vi "StateSpace_WalkThrough_Example.vi"() -> ()   [LabVIEW 2019]
uses:
  <vilib>/Rock Robotics/WPI/ThirdParty/JAS_Junk/TrajLib/TypeDef/LINEAR_SYSTEM.ctl
  <vilib>/Analysis/Matrix/Datatypes/RealMatrix.ctl
  <vilib>/Rock Robotics/WPI/ThirdParty/JAS_Junk/TrajLib/TypeDef/DCMOTOR.CTL
  <vilib>/Rock Robotics/WPI/ThirdParty/JAS_Junk/TrajLib/TypeDef/LINEAR_QUADRATIC_REGULATOR.ctl
  <vilib>/Rock Robotics/WPI/ThirdParty/JAS_Junk/TrajLib/TypeDef/KALMAN_FILTER.ctl
  <vilib>/Rock Robotics/WPI/ThirdParty/JAS_Junk/TrajLib/TypeDef/LINEAR_SYSTEM_LOOP.ctl
  <vilib>/Rock Robotics/WPI/ThirdParty/JAS_Junk/TrajLib/TypeDef/LINEAR_PLANT_INV_FF.ctl
  <vilib>/Rock Robotics/WPI/ThirdParty/JAS_Junk/TrajLib/TypeDef/FLYWHEEL_SIM.ctl
  <vilib>/Rock Robotics/WPI/ThirdParty/JAS_Junk/TrajLib/TypeDef/LINEAR_SYSTEM_SIM.ctl
  <vilib>/Rock Robotics/WPI/ThirdParty/JAS_Junk/TrajLib/Enum/DCMOTOR_TYPES_ENUM.ctl
  <vilib>/Rock Robotics/WPI/ThirdParty/JAS_Junk/TrajLib/DCMotor_GetCIM.vi
  <vilib>/Rock Robotics/WPI/ThirdParty/JAS_Junk/TrajLib/DCMotor_GetAndymark9015.vi
  <vilib>/Rock Robotics/WPI/ThirdParty/JAS_Junk/TrajLib/DCMotor_GetAndymarkRs775_125.vi
  <vilib>/Rock Robotics/WPI/ThirdParty/JAS_Junk/TrajLib/DCMotor_GetBag.vi
  <vilib>/Rock Robotics/WPI/ThirdParty/JAS_Junk/TrajLib/DCMotor_GetBanebotsRs550.vi
  <vilib>/Rock Robotics/WPI/ThirdParty/JAS_Junk/TrajLib/DCMotor_GetBanebotsRs775.vi
  <vilib>/Rock Robotics/WPI/ThirdParty/JAS_Junk/TrajLib/DCMotor_GetFalcon500.vi
  <vilib>/Rock Robotics/WPI/ThirdParty/JAS_Junk/TrajLib/DCMotor_GetMiniCIM.vi
  <vilib>/Rock Robotics/WPI/ThirdParty/JAS_Junk/TrajLib/DCMotor_GetNEO.vi
  <vilib>/Rock Robotics/WPI/ThirdParty/JAS_Junk/TrajLib/DCMotor_GetNEO550.vi
  <vilib>/Rock Robotics/WPI/ThirdParty/JAS_Junk/TrajLib/DCMotor_GetRomiBuiltIn.vi
  <vilib>/Rock Robotics/WPI/ThirdParty/JAS_Junk/TrajLib/DCMotor_GetVex775Pro.vi
  <vilib>/Rock Robotics/WPI/ThirdParty/JAS_Junk/TrajLib/MatBuilder_Create.vi
  <vilib>/Rock Robotics/WPI/ThirdParty/JAS_Junk/TrajLib/LinearSystem_New.vi
  <vilib>/Rock Robotics/WPI/ThirdParty/JAS_Junk/TrajLib/MatrixHelper_Zero.vi
  <vilib>/Rock Robotics/WPI/ThirdParty/JAS_Junk/TrajLib/MatBuilder_Fill.vi
  <vilib>/Rock Robotics/WPI/ThirdParty/JAS_Junk/TrajLib/Matrix_Ident.vi
  <vilib>/Rock Robotics/WPI/ThirdParty/JAS_Junk/TrajLib/LinearFilter_ResetToValue.vi
  <vilib>/Rock Robotics/WPI/ThirdParty/JAS_Junk/TrajLib/LinearFilter_Calculate.vi
  <vilib>/Rock Robotics/WPI/ThirdParty/JAS_Junk/TrajLib/DCMotor_New.vi
  <vilib>/Rock Robotics/WPI/ThirdParty/JAS_Junk/TrajLib/VI/Units_RotationsPerMinuteToRadiansPerSecond.vi
  <vilib>/Rock Robotics/WPI/ThirdParty/JAS_Junk/TrajLib/MatrixHelper_CoerceSize.vi
  <vilib>/Analysis/7linalg.llb/Create Special Matrix.vi
  <vilib>/Analysis/7linalg.llb/Create Special Real Matrix.vi
  <vilib>/Rock Robotics/WPI/ThirdParty/JAS_Junk/TrajLib/LinearFilter_MovingAverage.vi
  <vilib>/Rock Robotics/WPI/ThirdParty/JAS_Junk/TrajLib/LinearFilter_LowPassBW1.vi
  <vilib>/Rock Robotics/WPI/ThirdParty/JAS_Junk/TrajLib/LinearFilter_LowPassBW2.vi
  <vilib>/Rock Robotics/WPI/ThirdParty/JAS_Junk/TrajLib/LinearFilter_HighPassBW1.vi
  <vilib>/Rock Robotics/WPI/ThirdParty/JAS_Junk/TrajLib/LinearFilter_HighPassBW2.vi
  <vilib>/Rock Robotics/WPI/ThirdParty/JAS_Junk/TrajLib/Trajectory_Library.lvlib
  <vilib>/Analysis/Matrix/NI_Matrix.lvlib
panel:
  out "Linear System Loop":T1
  in  "Tab Control":T7(tab)
  out "m_flywheelPlant":T6
  out "Error\nSize Coerced":bool
  out "Shooter Motor":T8 {"Jr_KgM2" format="%13.5p"; "L_H" format="%13.5p"; "Kt_NMPerAmp" format="%13.5p"; "KvINV_RadPerSecPerVolt" format="%13.5p"; "R_Ohms" format="%13.5p"; "FreeSpeed_RadPerSec" format="%13.5p"; "FreeCurrent_Amps" format="%13.5p"; "StallCurrent_Amps" format="%13.5p"; "StallTorque_NM" format="%13.5p"; "nominalVoltage_Volts" format="%13.5p"}
  out "m_flywheelPlant_ALT":T6
  out "KalmanFilter":T5
  out "Kalman Creation Error":errorcluster
  out "LinearQuadraticRegulator":T2
  out "LQR Creation Error":bool
  out "Linear System Loop":T1
  out "LinSysLoop_Error":bool
  out "CO, Filtered Voltage, Filtered Current Chart":T9(graph)
  out "Filtereed Battery Voltage":dbl format="%20.3f"
  out "Filtereed Current (Amps)":dbl format="%20.3f"
  in  "Shooter \nOn/Off":bool
  out "Encoder Speed\nRad/Sec":dbl(slide) scale=0.0..300.0
  out "Speed \nRad/Sec":dbl format="%16.1f"
  out "Execution\nError":bool
  out "Kalman Filtered\nSpeed Rad/Sec":dbl format="%16.1f"
  out "SP, PV Chart":T9(graph)
  out "Motor Dmd CO":dbl format="%20.3f"
  out "Speed Setpoint\nRad/Sec":dbl format="%16.1f"
  in  "Set Point\nRad/Sec 2":dbl(slide) scale=0.0..300.0
  out "m_FlyWheelSim":T10 {"GearBox"."Jr_KgM2" format="%13.5p"; "GearBox"."L_H" format="%13.5p"; "GearBox"."Kt_NMPerAmp" format="%13.5p"; "GearBox"."KvINV_RadPerSecPerVolt" format="%13.5p"; "GearBox"."R_Ohms" format="%13.5p"; "GearBox"."FreeSpeed_RadPerSec" format="%13.5p"; "GearBox"."FreeCurrent_Amps" format="%13.5p"; "GearBox"."StallCurrent_Amps" format="%13.5p"; "GearBox"."StallTorque_NM" format="%13.5p"; "GearBox"."nominalVoltage_Volts" format="%13.5p"}
  # "<States,1>"
  # "<FUTURE --- CLAMP TYPE -- For now\nuse Normalize>"
  # "Steady State Gain  \n<States,Outputs>"
  # "State Estimate <Statess,1>"
  # "<States,States>"
  # "<States,Inputs>"
  # "<Outputs,States>"
  # "<Outputs,Inputs>"
  # "<States,1>"
  # "<Inputs,1>"
  # "<States,Inputs>"
  # "<States,States>"
  # "Ref State <States,1>"
  # "Comp and capped \noutput <Inputs,1>"
  # "Controller gain\n<Inputs,States>"
  # "The \"plant\" holds a state-space model of our flywheel. This system has the following properties:\n\n   -  States: [velocity], in radians per second.\n   -  Inputs (what we can \"put in\"): [voltage], in volts.\n   -  Outputs (what we can measure): [velocity], in radians per second.\n\nThere are also constants describing how the system behaves.  For our system these are:\n    Kv ---  Volts per (radian per second)\n    Ka --- Volts per (radian per second squared)\n\n One way the Kv and Ka constants can be found by using the FRC Characterization toolsuite.  \n\nNOTE:\n    Constants were changed to create a more realistic simulation."
  # "<States,States>"
  # "<States,Inputs>"
  # "<Outputs,States>"
  # "<Outputs,Inputs>"
  # "Another way to create a linear system is to use the \"helpers\" available for certain types of systems.\n\nThis uses the following contants:\n   -  DcMotor   --  model cooeficients for a pariticular number of a particular model of motor.\n   -  kFlywheelMomentOfInertia = 0.00032    --    kg * m^2\n   -  kFlywheelGearing = 1.0    --  Reduction between motors and encoder, \n                                     as output over input. If the flywheel spins slower than\n                                     the motors, this number should be greater than one.\n\nThe plant holds a state-space model of our flywheel. This system has the following properties:\n   -  States: [velocity], in radians per second.\n   -  Inputs (what we can \"put in\"): [voltage], in volts.\n   -  Outputs (what we can measure): [velocity], in radians per second.\n\nNOTE:\n    Constants were changed to create a more realistic simulation."
  # "<States,States>"
  # "<States,Inputs>"
  # "<Outputs,States>"
  # "<Outputs,Inputs>"
  # "Create a Kalman Filter.  This filters the measurment data, by using the \nLinear System model and how accurate we think the model and \nmeasurements are.  \n\nThe parameters are:\n   - States  --  Number of states in the Linear System\n   - Outputs  --  Number of outputs in the Linear System.\n   - State Std Dev  --  How accurate we think our model is\n   - Measurement Std Dev  --  How accurate we think our encoder data is\n   - dtSeconds  --  How often the control loop will be executed.\n\nNOTE:\n    Constants were changed to create a more realistic simulation."
  # "Steady State Gain  \n<States,Outputs>"
  # "State Estimate <Statess,1>"
  # "<States,States>"
  # "<States,Inputs>"
  # "<Outputs,States>"
  # "<Outputs,Inputs>"
  # "Create the Linear Quadratic Controller.   This takes the measurement input (filtered or not), the desired\nsetpoint (Next R) and calculates the desired motor demand output  U. (Linear System Input) .\n\nCreation of the Linear Quadratic Controller (LQR) takes the following inputs:\n\n   - The Linear System model\n   - Qelms  --  Velocity error tolerance, in radians per second. Decrease\n                         this to more heavily penalize state excursion, or make the controller \n                          behave more aggressively.\n   - Relms  --  Control effort (voltage) tolerance. Decrease this to more\n                        heavily penalize control effort, or make the controller less \n                        aggressive. 12 is a good starting point because that is the \n                        (approximate) maximum voltage of a battery.\n   - dtSeconds  --  Nominal time between loops."
  # "Ref State <States,1>"
  # "Comp and capped \noutput <Inputs,1>"
  # "Controller gain\n<Inputs,States>"
  # "Put everything created so far together into\na Linear System Loop.  This is a convience\nfunction used to help simplify run-time\nexecution."
  # "<States,1>"
  # "<FUTURE --- CLAMP TYPE -- For now\nuse Normalize>"
  # "Steady State Gain  \n<States,Outputs>"
  # "State Estimate <Statess,1>"
  # "<States,States>"
  # "<States,Inputs>"
  # "<Outputs,States>"
  # "<Outputs,Inputs>"
  # "<States,1>"
  # "<Inputs,1>"
  # "<States,Inputs>"
  # "<States,States>"
  # "Ref State <States,1>"
  # "Comp and capped \noutput <Inputs,1>"
  # "Controller gain\n<Inputs,States>"
  # "This subVI is called from a loop that runs every\n20 milliseconds.  The single execution loop with\nshift register in the subVI allows the linear system\nloop state to be saved between calls."
  # "The execution steps are:\n\n1) Set the speed setpoint.\n\n2) Feed the current encoder speed measurement to the \n    controller\n\n3) Execute \"Correct\".  In this step the Kalman filter updates \n    the system state vector with the filtered encoder data.\n\n4) Execute \"Predict\".  This updates the LQR controller to \n    generate new voltage commands and use the voltages \n    to predict the next state with out Kalman filter.\n\n5) Get the desirec motor demand.  This is volts.  It needs \n    to be scaled to +/- 1.0 by dividing by 12.0 to send to the \n    motor controller."
  # "This simulates the Flywheel so the encoder speed can\nbe obtained for this example."
  # "<States, 1>"
  # "<Outputs, 1>"
  # "<Inputs, 1>"
  # "<Outputs, 1>"
  # "<States,States>"
  # "<States,Inputs>"
  # "<Outputs,States>"
  # "<Outputs,Inputs>"
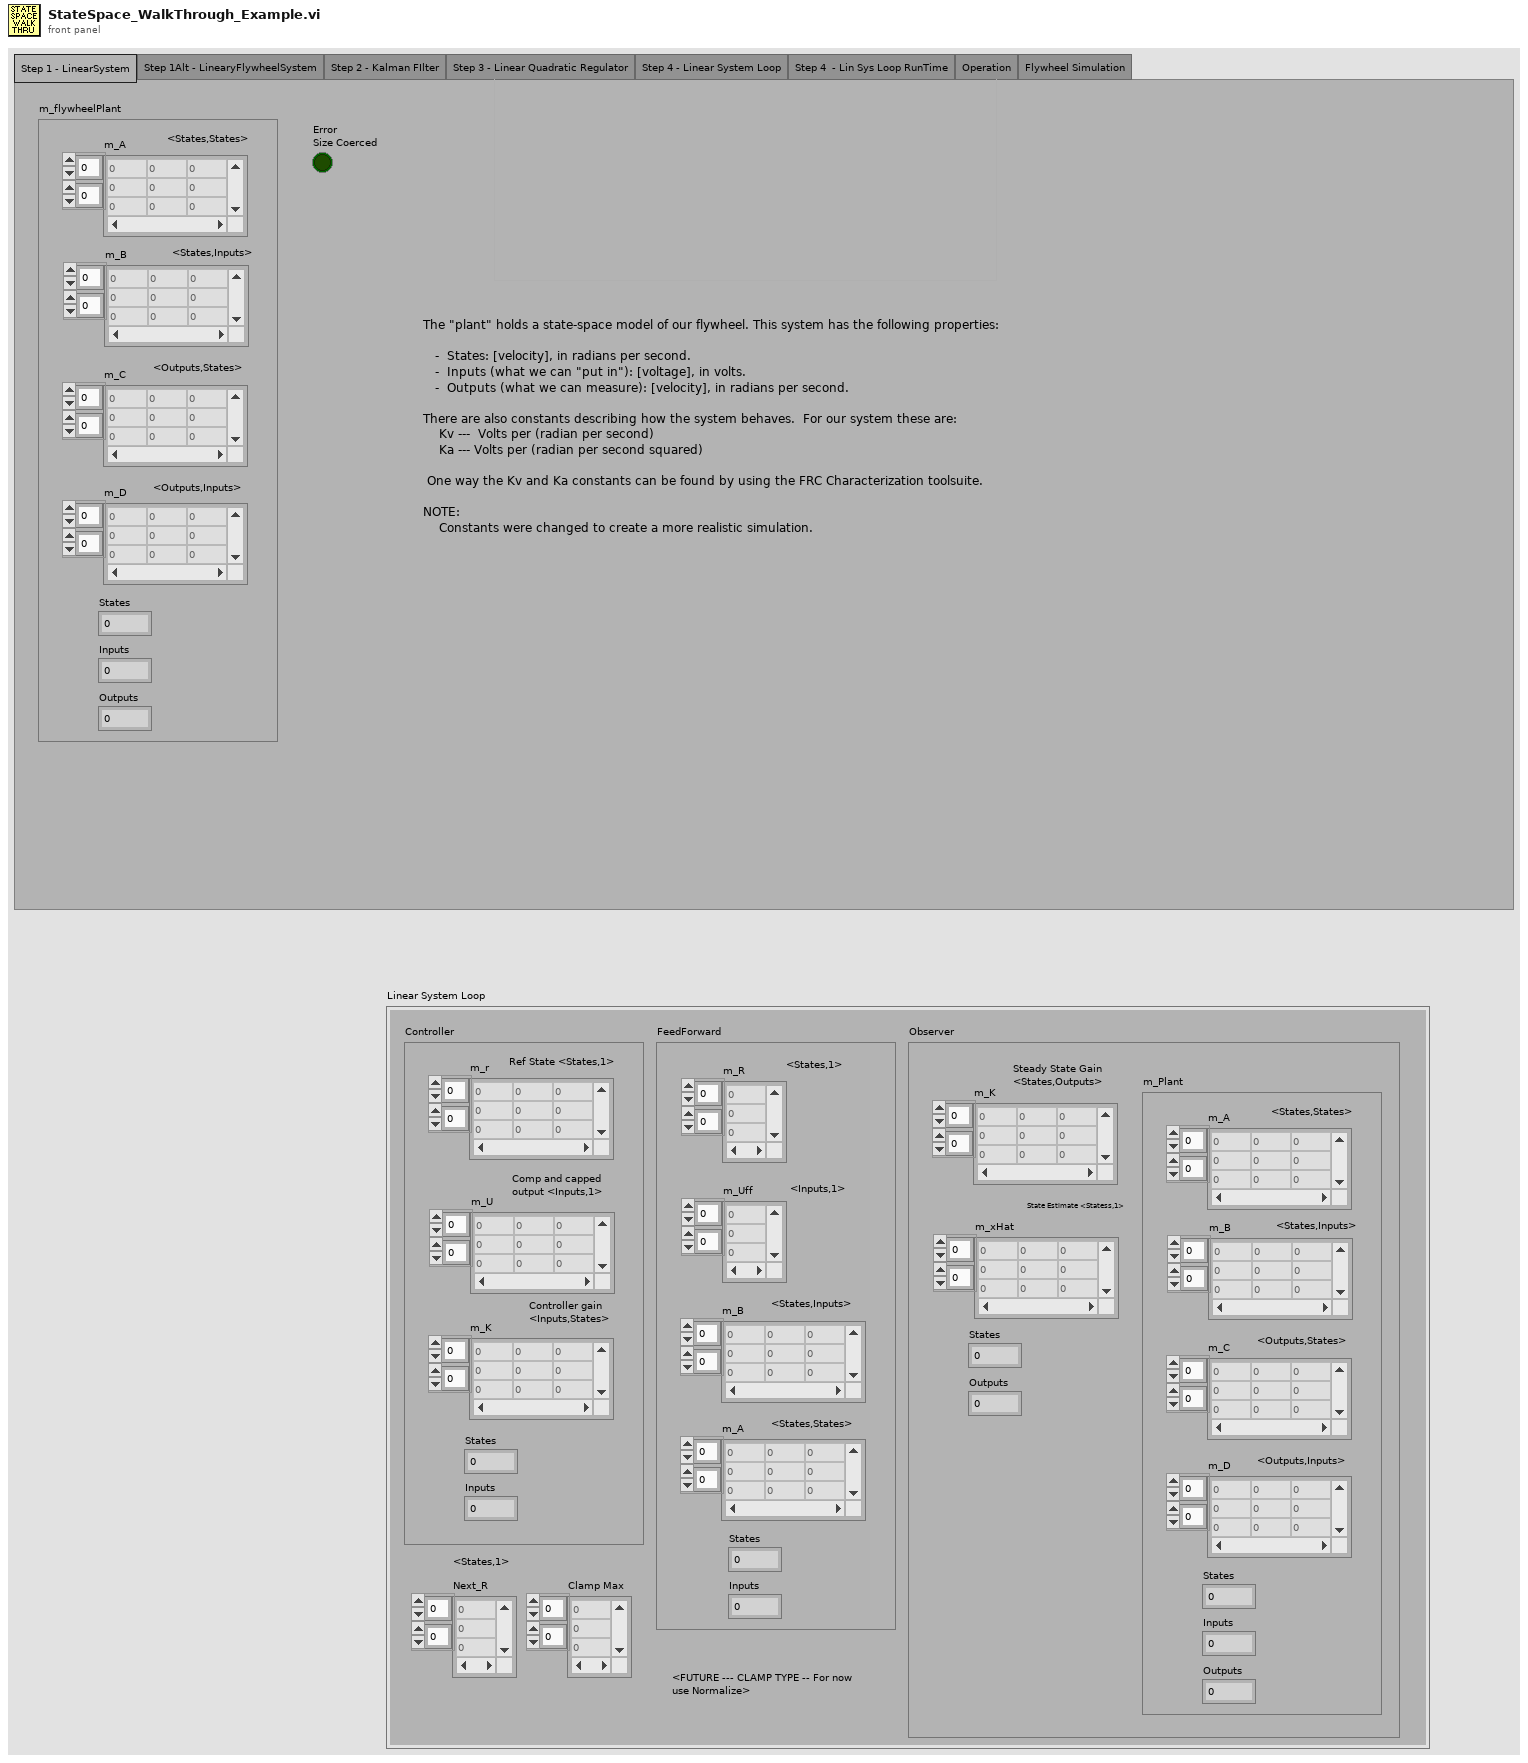
[diagram p1: front panel]
types:
  T1 = typedef "Trajectory_Library.lvlib/LINEAR_SYSTEM_LOOP.ctl" = cluster{"Controller":T2, "FeedForward":T4, "Observer":T5, "Next_R":T3, "Clamp Max":T3}
  T2 = typedef "Trajectory_Library.lvlib/LINEAR_QUADRATIC_REGULATOR.ctl" = cluster{"m_r":T3, "m_U":T3, "m_K":T3, "States":i32, "Inputs":i32}
  T3 = typedef "NI_Matrix.lvlib/RealMatrix.ctl" = dbl[][]
  T4 = typedef "Trajectory_Library.lvlib/LINEAR_PLANT_INV_FF.ctl" = cluster{"m_R":T3, "m_Uff":T3, "m_B":T3, "m_A":T3, "States":i32, "Inputs":i32}
  T5 = typedef "Trajectory_Library.lvlib/KALMAN_FILTER.ctl" = cluster{"m_K":T3, "m_xHat":T3, "States":i32, "Outputs":i32, "m_Plant":T6}
  T6 = typedef "Trajectory_Library.lvlib/LINEAR_SYSTEM.ctl" = cluster{"m_A":T3, "m_B":T3, "m_C":T3, "m_D":T3, "States":i32, "Inputs":i32, "Outputs":i32}
  T7 = enum32{"Step 1 - LinearSystem", "Step 1Alt - LinearyFlywheelSystem", "Step 2 - Kalman FIlter", "Step 3 - Linear Quadratic Regulator", "Step 4 - Linear System Loop", "Step 4  - Lin Sys Loop RunTime", "Operation", "Flywheel Simulation"}
  T8 = typedef "Trajectory_Library.lvlib/DCMOTOR.CTL" = cluster{"nominalVoltage_Volts":dbl, "StallTorque_NM":dbl, "StallCurrent_Amps":dbl, "FreeCurrent_Amps":dbl, "FreeSpeed_RadPerSec":dbl, "R_Ohms":dbl, "KvINV_RadPerSecPerVolt":dbl, "Kt_NMPerAmp":dbl, "L_H":dbl, "Jr_KgM2":dbl}
  T9 = cluster{"upper limit":dbl, "Real Matrix Element":dbl, "Real Matrix Element":dbl}
  T10 = typedef "Trajectory_Library.lvlib/FLYWHEEL_SIM.ctl" = cluster{"LinearSystemSim":T11, "GearBox":T8, "Gearing":dbl}
  T11 = typedef "Trajectory_Library.lvlib/LINEAR_SYSTEM_SIM.ctl" = cluster{"m_Plant":T6, "m_X":T3, "m_Y":T3, "m_U":T3, "MeasureStdDev":T3}
  T12 = typedef "Trajectory_Library.lvlib/DCMOTOR_TYPES_ENUM.ctl" = enum16{"CIM", "AndyMark 9015", "Andy Mark RS 775 125", "Bag", "BaneBots RS 550", "BaneBots RS 775", "Falcon 500", "Mini CIM", "NEO", "NEO 550", "Romi BuiltIn", "Vex 775 Pro"}
  T13 = enum16{"Moving Average", "Low Pass 1st Order Butterworth", "Low Pass 2nd Order Butterworth", "High Pass 1st Order Butterworth", "High Pass 2nd Order Butterworth"}
  T14 = cluster{"Speed Rad/Sec\nPV":dbl, "Filtered PV":dbl, "R0_C0":dbl}
  T15 = cluster{"Motor Dmd CO":dbl, "Output":dbl, "Output":dbl}
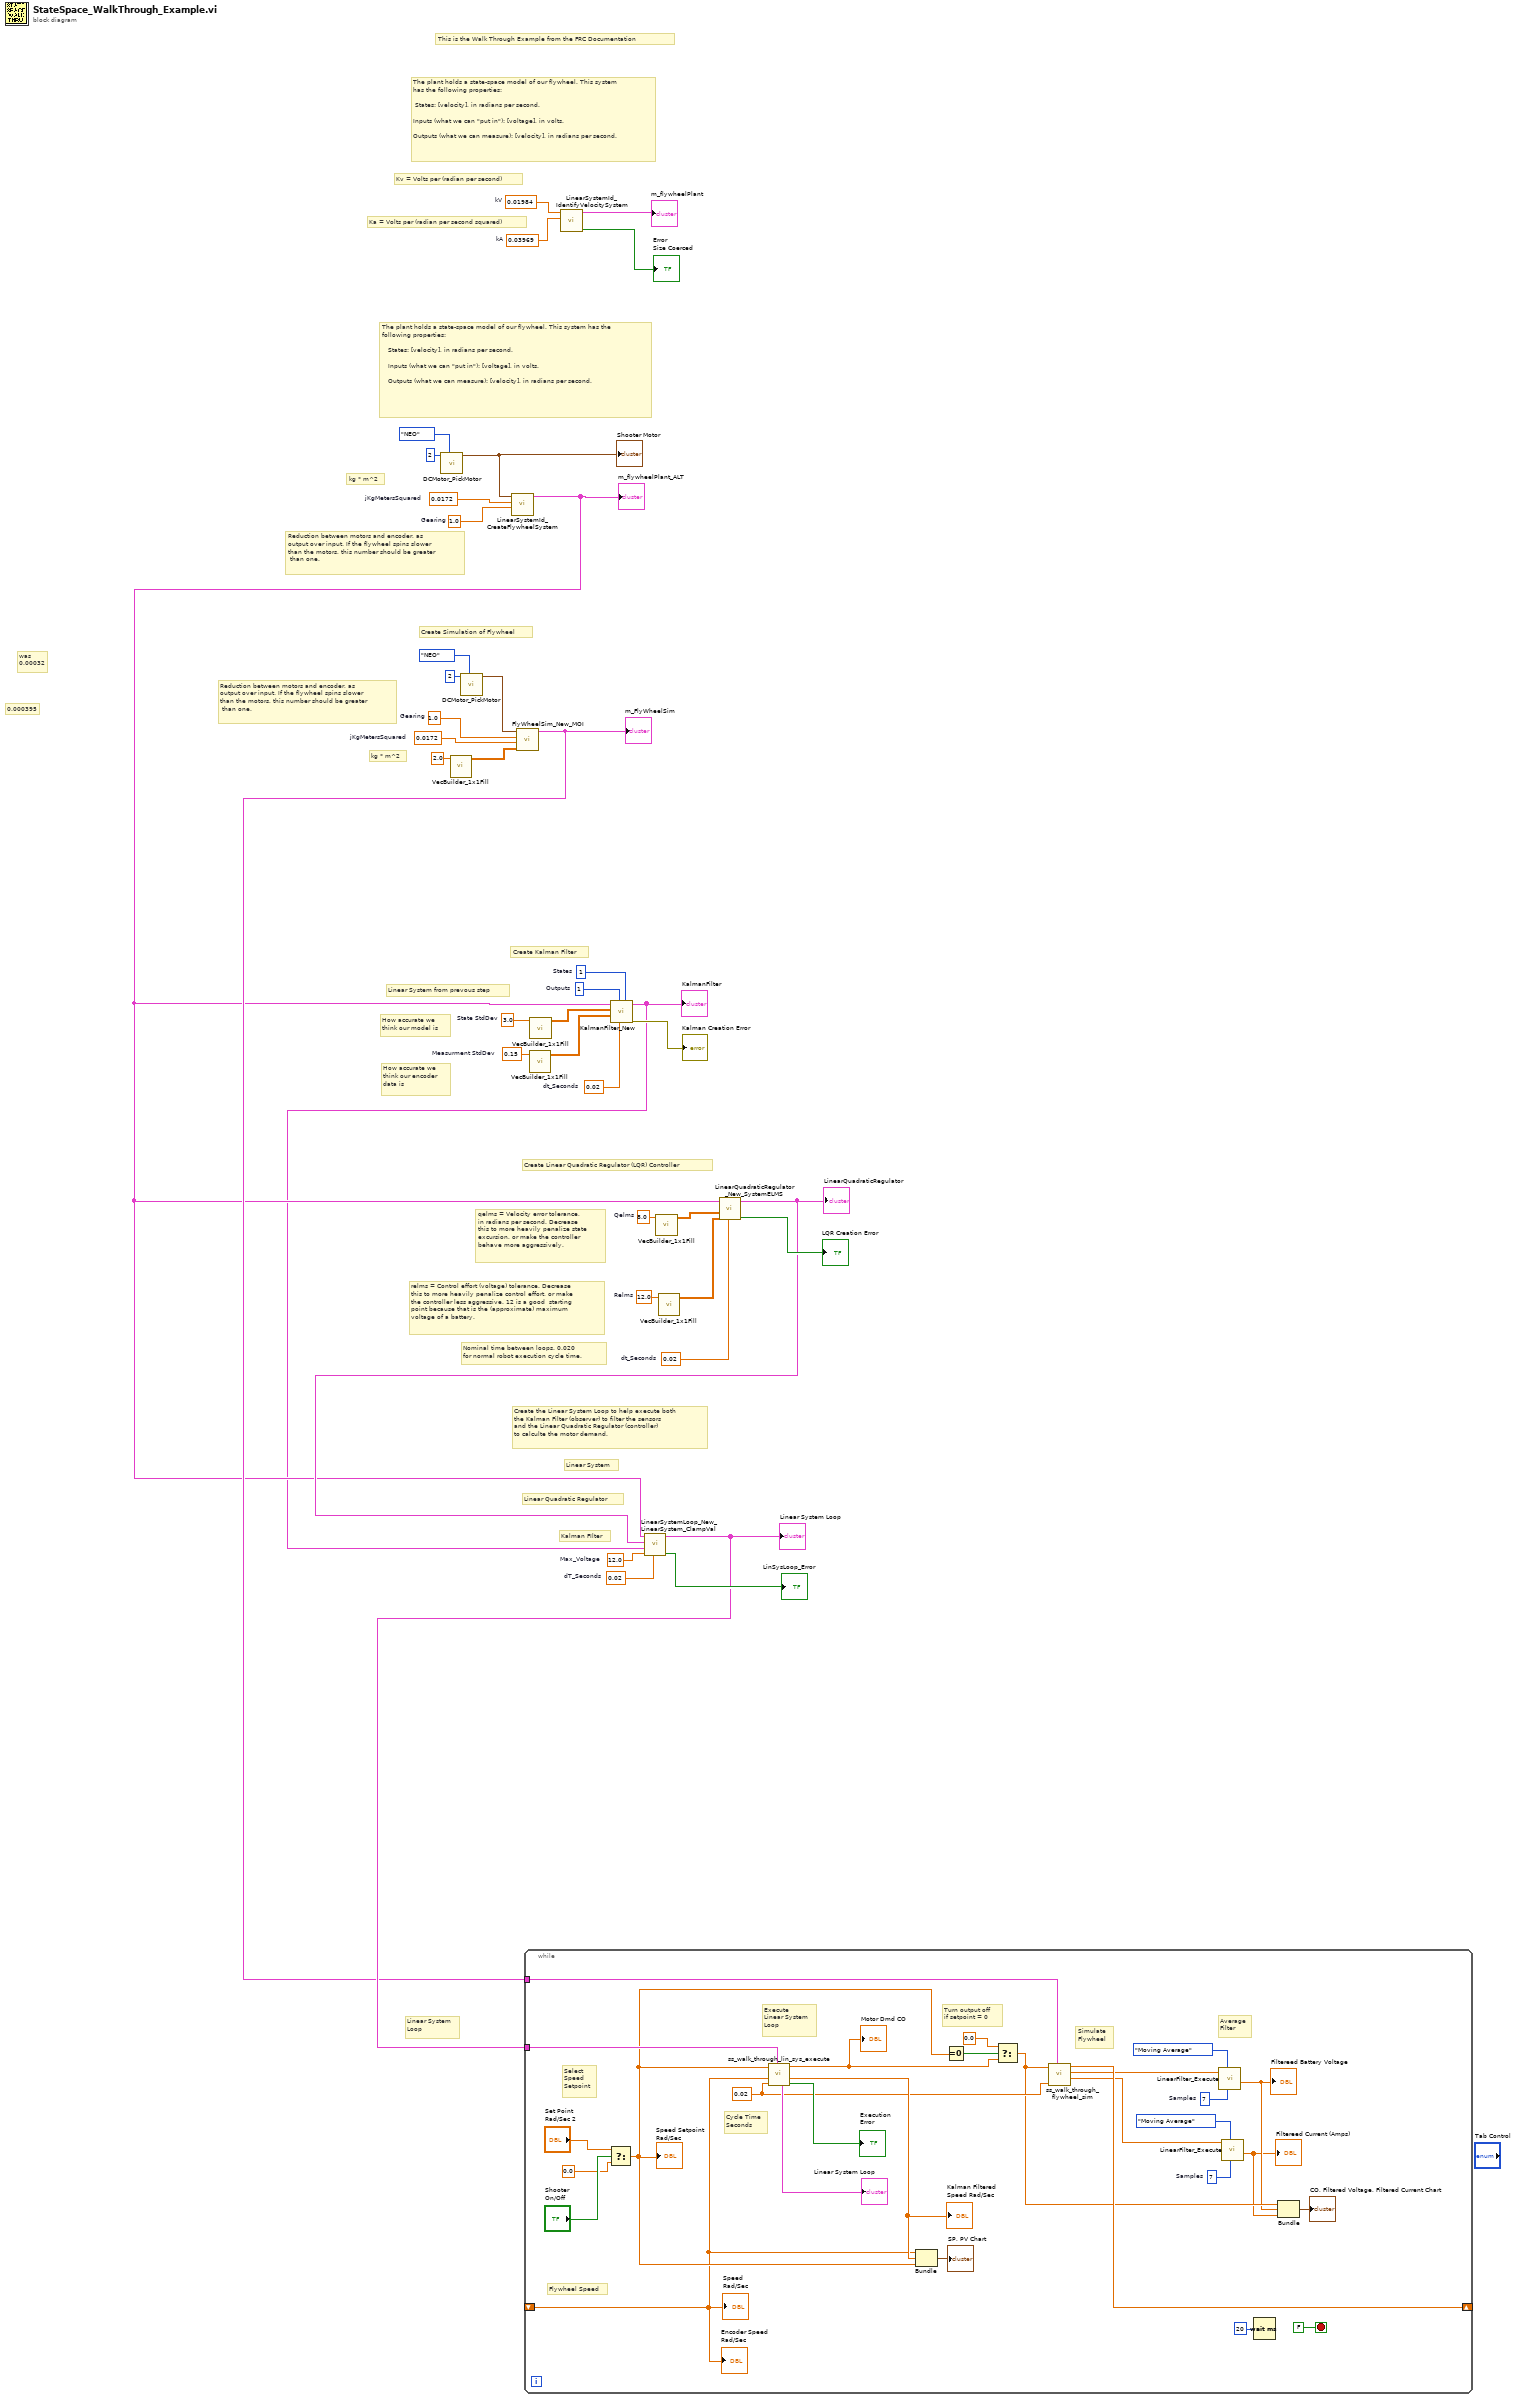
[diagram p0: block diagram]
diagram:
  w6 = 0.0172  # jKgMetersSquared
  w5 = 1.0  # Gearing
  w14 = 0.0172  # jKgMetersSquared
  w19 = 0.02  # dT_Seconds
  w20 = 12.0  # Max_Voltage
  w24 = 0.02  # dt_Seconds
  w25 = 0.15  # Measurment StdDev
  w26 = 3.0  # State StdDev
  w27 = 1  # States
  w28 = 1  # Outputs
  w32 = 12.0  # Relms
  w33 = 8.0  # Qelms
  w30 = 0.02  # dt_Seconds
  w17 = 1.0  # Gearing
  w37 = 0.03969  # kA
  w38 = 0.01984  # kV
  # "Linear System\nLoop"
  # "0.000395"
  # "was\n0.00032"
  # "Create the Linear System Loop to help execute both \nthe Kalman Filter (observer) to filter the sensors\nand the Linear Quadratic Regulator (controller) \nto calculte the motor demand."
  # "Nominal time between loops. 0.020 \nfor normal robot execution cycle time."
  # "relms = Control effort (voltage) tolerance. Decrease \nthis to more heavily penalize control effort, or make \nthe controller less aggressive. 12 is a good  starting \npoint because that is the (approximate) maximum \nvoltage of a battery."
  # "Create Linear Quadratic Regulator (LQR) Controller"
  # "qelms = Velocity error tolerance, \nin radians per second. Decrease\nthis to more heavily penalize state \nexcursion, or make the controller \nbehave more aggressively."
  # "Create Kalman Filter"
  # "How accurate we \nthink our encoder\ndata is"
  # "How accurate we \nthink our model is"
  # "Reduction between motors and encoder, as \noutput over input. If the flywheel spins slower \nthan the motors, this number should be greater\n than one."
  # "kg * m^2"
  # "Reduction between motors and encoder, as \noutput over input. If the flywheel spins slower \nthan the motors, this number should be greater\n than one."
  # "kg * m^2"
  # "The plant holds a state-space model of our flywheel. This system \nhas the following properties:\n \n States: [velocity], in radians per second.\n  \nInputs (what we can \"put in\"): [voltage], in volts.\n  \nOutputs (what we can measure): [velocity], in radians per second."
  # "Ka = Volts per (radian per second squared)"
  # "Kv = Volts per (radian per second)"
  # "This is the Walk Through Example from the FRC Documentation"
  # "Kalman FIlter"
  # "Linear Quadratic Regulator"
  # "Linear System"
  # "Linear System from prevous step"
  # "Create Simulation of Flywheel"
  # "The plant holds a state-space model of our flywheel. This system has the \nfollowing properties:\n\n   States: [velocity], in radians per second.\n\n   Inputs (what we can \"put in\"): [voltage], in volts.\n\n   Outputs (what we can measure): [velocity], in radians per second."
  n1 = call <vilib>:"DCMotor_PickMotor.vi"("DCMOTOR_TYPES"=DCMOTOR_TYPES_ENUM."NEO", "Num Motors"=2) -> ("DCMOTOR"=w12:T8)  [unwired: 9 in]
  "Shooter Motor" <- w12
  n2 = call <vilib>:"VecBuilder_1x1Fill.vi"("R0_C0"=2.0) -> ("output matrix"=w16:T3)  [unwired: 10 in]
  n3 = call <vilib>:"DCMotor_PickMotor.vi"("DCMOTOR_TYPES"=DCMOTOR_TYPES_ENUM."NEO", "Num Motors"=2) -> ("DCMOTOR"=w8:T8)  [unwired: 9 in]
  n4 = call <vilib>:"LinearSystemId_CreateFlywheelSystem.vi"("G"=w17, "jKgMetersSquared"=w14, "DCMOTOR"=w12) -> ("Linearsystem"=w2:T6)  [unwired: 7 in, 1 out]
  "m_flywheelPlant_ALT" <- w2
  n5 = call <vilib>:"FlyWheelSim_New_MOI.vi"("MeasurementStdDev"=w16, "jKgMetersSquared"=w6, "Gearing"=w5, "GearBox"=w8) -> ("FlyWheelSim"=w3:T10)  [unwired: 6 in, 1 out]
  "m_FlyWheelSim" <- w3
  n6 = call <vilib>:"VecBuilder_1x1Fill.vi"("R0_C0"=w25) -> ("output matrix"=w22:T3)  [unwired: 10 in]
  n7 = call <vilib>:"VecBuilder_1x1Fill.vi"("R0_C0"=w26) -> ("output matrix"=w23:T3)  [unwired: 10 in]
  n8 = call <vilib>:"LinearSystemId_IdentifyVelocitySystem.vi"("kA"=w37, "kV"=w38) -> ("Size Coerced"=→"Error\nSize Coerced":bool, "Linearsystem"=→"m_flywheelPlant":T6)  [unwired: 8 in]
  n9 = call <vilib>:"KalmanFilter_New.vi"("States"=w27, "dt_Seconds"=w24, "Outputs"=w28, "MeasurementStdDevs"=w22, "StateStdDevs"=w23, "Plant"=w2) -> ("Error"=→"Kalman Creation Error":errorcluster, "KalmanFilter"=w1:T5)  [unwired: 4 in]
  "KalmanFilter" <- w1
  n10 = call <vilib>:"VecBuilder_1x1Fill.vi"("R0_C0"=w33) -> ("output matrix"=w31:T3)  [unwired: 10 in]
  n11 = call <vilib>:"VecBuilder_1x1Fill.vi"("R0_C0"=w32) -> ("output matrix"=w29:T3)  [unwired: 10 in]
  n12 = call <vilib>:"LinearQuadraticRegulator_New_SystemELMS.vi"("dt_Seconds"=w30, "Relms"=w29, "Qelms"=w31, "LINEARSYSTEM"=w2) -> ("Error"=→"LQR Creation Error":bool, "LinearQuadraticRegulator"=w7:T2)  [unwired: 6 in]
  "LinearQuadraticRegulator" <- w7
  n13 = call <vilib>:"LinearSystemLoop_New_LinearSystem_ClampVal.vi"("dT_Seconds"=w19, "Max_Voltage"=w20, "Observer"=w1, "Controller"=w7, "Plant"=w2) -> ("Error"=→"LinSysLoop_Error":bool, "Linear System Loop"=w4:T1)  [unwired: 5 in]
  "Linear System Loop" <- w4
  n14 = while {
    tunnel: w4 -> [w59]
    tunnel: w3 -> [w54]
    shift-right: [w51] -> _
    shift-left: _ -> [w50]
    stop <- FALSE stop-if-true
    w43 = 7  # Samples
    w46 = 7  # Samples
    w53 = 0.02 ("dT_Seconds")
    # "Average\nFilter"
    # "Flywheel Speed"
    # "Simulate \nFlywheel"
    # "Turn output off\nif setpoint = 0"
    # "Cycle Time\nSeconds"
    # "Select\nSpeed\nSetpoint"
    # "Execute\nLinear System\nLoop"
    n15 = Select(t="Set Point\nRad/Sec 2", s="Shooter \nOn/Off", f=0.0 ("R0_C0")) -> (s? t:f=w52:dbl)
    "Speed Setpoint\nRad/Sec" <- w52
    n16 = call "ss_walk_through_lin_sys_execute.vi"("init Linear \nSystem\nLoop"=w59, "Cycle Time \nSeconds"=w53, "Process Variable PV"=w50, "Setpoint SP"=w52) -> ("Error"=→"Execution\nError":bool, "Filtered PV"=w58:dbl, "Motor Dmd CO"=w49:dbl, "out Linear \nSystem Loop"=→"Linear System Loop":T1)  [unwired: 4 in]
    "Kalman Filtered\nSpeed Rad/Sec" <- w58
    "Motor Dmd CO" <- w49
    n17 = Bundle("Speed Rad/Sec\nPV"=w50, "Filtered PV"=w58, "R0_C0"=w52) -> (→"SP, PV Chart":T14)  [unwired: 1 in]
    n18 = Equal To 0?(x=w52) -> (x = 0?=w63:bool)
    n19 = Select(t=0.0, s=w63, f=w49) -> (s? t:f=w47:dbl)
    n20 = call "ss_walk_through_flywheel_sim.vi"("init FlyWheelSim"=w54, "Cycle Time\nSeconds"=w53, "Motor Dmd\nCO"=w47) -> ("Current Amps"=w41:dbl, "Battery Voltage"=w44:dbl, "Speed Rad/Sec\nPV"=w51:dbl)  [unwired: 5 in, 1 out]
    n21 = call <vilib>:"LinearFilter_Execute.vi"("Samples"=w46, "Filter Type"=T13."Moving Average", "Input"=w44) -> ("Output"=w40:dbl)  [unwired: 7 in, 1 out]
    "Filtereed Battery Voltage" <- w40
    n22 = call <vilib>:"LinearFilter_Execute.vi"("Samples"=w43, "Filter Type"=T13."Moving Average", "Input"=w41) -> ("Output"=w39:dbl)  [unwired: 7 in, 1 out]
    "Filtereed Current (Amps)" <- w39
    n23 = Wait (ms)(milliseconds to wait=u32 20) -> ()  [unwired: 1 out]
    n24 = Bundle("Motor Dmd CO"=w47, "Output"=w40, "Output"=w39) -> (→"CO, Filtered Voltage, Filtered Current Chart":T15)  [unwired: 1 in]
    "Encoder Speed\nRad/Sec" <- w50
    "Speed \nRad/Sec" <- w50
  }
